vi "8-bit video export-AVI initialise split file.vi"(8 "error in":errorcluster, 9 "RGB image ref in":T1, 11 "AVI modes refs":T2) -> (0 "error out":errorcluster, 3 "AVI modes refs":T2)   [LabVIEW 2020]
uses:
  Typedefs/8-bit video export AVI modes cluster.ctl
  <vilib>/vision/Avi1.llb/AviRefnum.ctl
  <vilib>/vision/Avi.llb/IMAQ AVI2 Refnum.ctl
  <vilib>/vision/Image Controls.llb/IMAQ Image.ctl
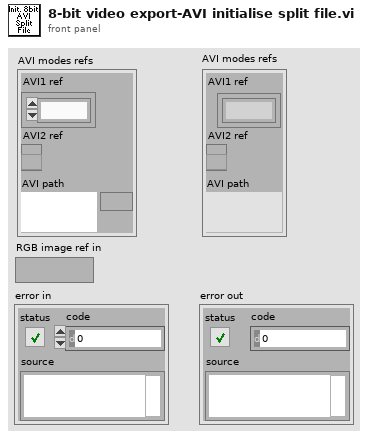
[diagram p1: front panel]
types:
  T1 = typedef "IMAQ Image.ctl" = refnum<image>
  T2 = typedef "8-bit video export AVI modes cluster.ctl" = cluster{"AVI1 ref":T3, "AVI2 ref":T4, "AVI path":path}
  T3 = typedef "AviRefnum.ctl" = refnum<k1>
  T4 = typedef "IMAQ AVI2 Refnum.ctl" = refnum<k20>
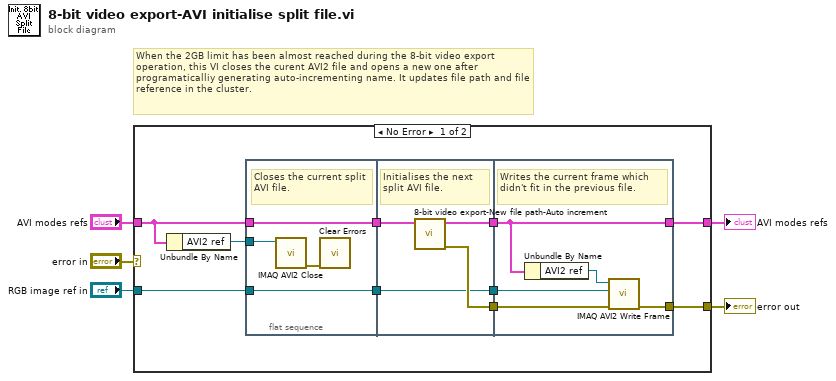
[diagram p0: block diagram]
diagram:
  # "When the 2GB limit has been almost reached during the 8-bit video export operation, this VI closes the curent AVI2 file and opens a new one after programaticalliy generating auto-incrementing name. It updates file path and file reference in the cluster."
  n1 = case shown="No Error" "error in" {
    selector: "error in" -> [_ w30]
    tunnel: [w15 w30] -> w4
    tunnel: "AVI modes refs" -> [w11 w29]
    tunnel: [w12 w29] -> w2
    tunnel: "RGB image ref in" -> [w8 _]
    frame No Error {
      n2 = Unbundle By Name(w11) -> ("AVI2 ref"=w14:T4)
      n3 = flat-sequence {
        tunnel: w14 -> [w18]
        tunnel: [w17] -> w13
        tunnel: w11 -> [w17]
        tunnel: w8 -> [w16]
        tunnel: [w16] -> w7
        tunnel: w13 -> [w22]
        tunnel: [w23] -> w10
        tunnel: [w21] -> w9
        tunnel: w7 -> [w20]
        tunnel: [w20] -> w6
        tunnel: [w25] -> w12
        tunnel: [w27] -> w15
        tunnel: w10 -> [w28]
        tunnel: w9 -> [w25]
        tunnel: w6 -> [w26]
        frame #0 {
          # "Closes the current split AVI file."
          n4 = call "IMAQ AVI2 Close"("AVI Refnum"=w18) -> ("error out"=w19:errorcluster)  [unwired: 10 in]
          n5 = call <vilib>:"Clear Errors.vi"("error in (no error)"=w19) -> ()  [unwired: 5 in, 2 out]
        }
        frame #1 {
          # "Initialises the next split AVI file."
          n6 = call "8-bit video export-New file path-Auto increment.vi"("AVI modes refs"=w22) -> ("error out"=w23:errorcluster, "AVI modes refs"=w21:T2)  [unwired: 9 in]
        }
        frame #2 {
          # "Writes the current frame which didn't fit in the previous file."
          n7 = Unbundle By Name(w25) -> ("AVI2 ref"=w24:T4)
          n8 = call "IMAQ AVI2 Write Frame"("error in (no error)"=w28, "Image"=w26, "AVI Refnum"=w24) -> ("error out"=w27:errorcluster)  [unwired: 6 in, 2 out]
        }
      }
    }
    frame Error {
    }
  }
  "error out" <- w4
  "AVI modes refs" <- w2
